vi "createIDstring_01.vi"(1 "DeviceID":i32, 2 "DateTime":timestamp) -> (0 "result string":string)   [LabVIEW 2010]
panel:
  # "12 YYYY-MM-DD hh:mm:ss microseconds"
  # "12 2012-07-17 19:00:02 373503.7"
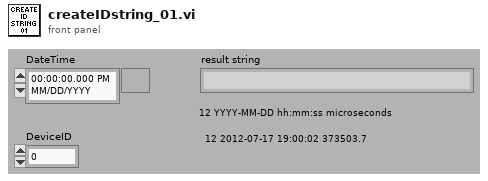
[diagram p1: front panel]
types:
  T1 = typedef "LVDateTimeRec.ctl" = cluster{"fractional second":dbl, "second":i32, "minute":i32, "hour":i32, "day of month":i32, "month":i32, "year":i32, "day of week":i32, "day of year":i32, "DST":i32}
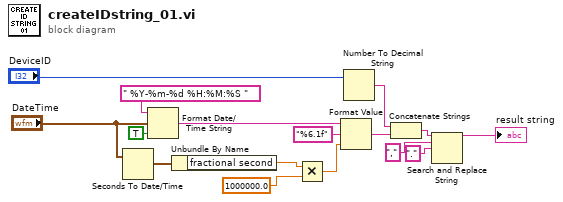
[diagram p0: block diagram]
diagram:
  n1 = Seconds To Date/Time(time stamp (now)="DateTime") -> (date time rec=w3:T1)  [unwired: 1 in]
  n2 = Format Date/Time String(time format string (%c)=" %Y-%m-%d %H:%M:%S ", seconds (now)="DateTime", UTC format=TRUE) -> (date/time string=w6:string)
  n3 = Unbundle By Name(w3) -> ("fractional second"=w4:dbl)
  n4 = Multiply(x=w4, y=1000000.0) -> (x*y=w7:dbl)
  n5 = Format Value(string ("")=w6, format string="%6.1f", value (0)=w7) -> (output string=w13:string)
  n6 = Number To Decimal String(number="DeviceID") -> (decimal integer string=w15:string)  [unwired: 1 in]
  n7 = Concatenate Strings(w15, w13) -> (w14:string)
  n8 = Search and Replace String(input string=w14, search string=",", replace string="." ("replace string (\"\")")) -> (result string=→"result string":string)  [unwired: 5 in, 3 out]
